vi "下拉列表-设置选项.vi"(1 "项名":string[](array[string]), 2 "error in (no error)":errorcluster caption="错误输入（无错误）", 3 "下拉列表":refnum<vi>) -> (0 "error out":errorcluster caption="错误输出")   [LabVIEW 2014]
doc: "该模板用于创建子VI。"
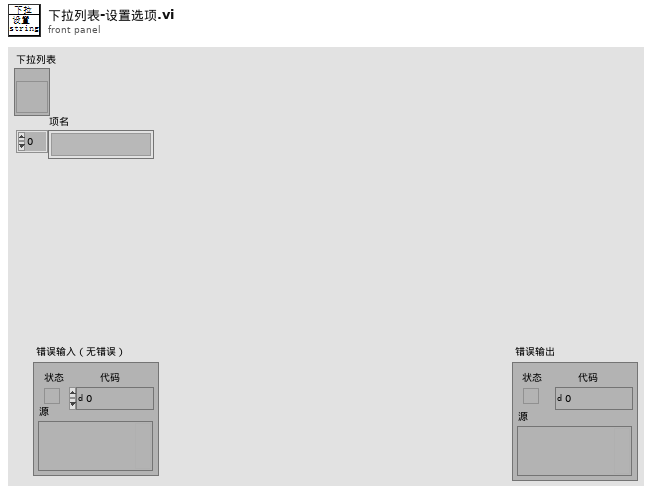
[diagram p1: front panel]
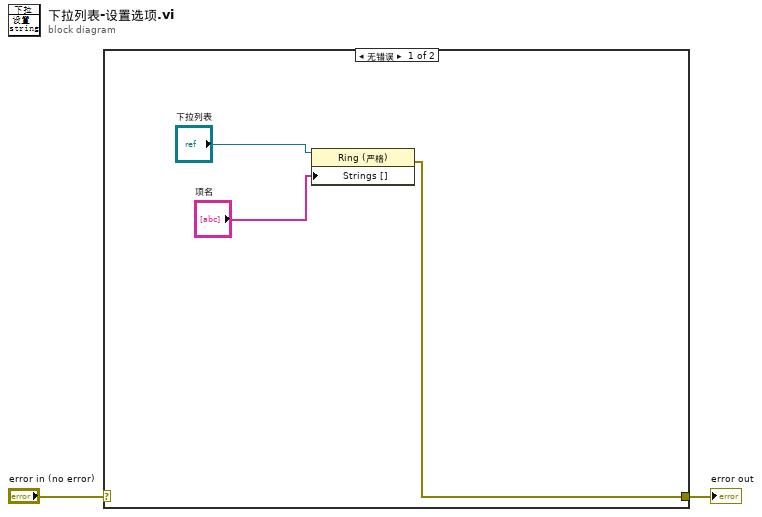
[diagram p0: block diagram]
diagram:
  n1 = case shown="无错误" "error in (no error)" {
    selector: "error in (no error)" -> [_ w6]
    tunnel: [w3 w6] -> w1
    frame No Error {
      n2 = property class="Ring (严格)"(reference="下拉列表", "Strings []"="项名") -> (error out=w3:errorcluster)  [unwired: 1 in, 1 out]
    }
    frame Error {
    }
  }
  "error out" <- w1
